vi "Contact closure.vi"(0 "Task In CC":refnum<k21>) -> ()   [LabVIEW 2016]
uses:
  <vilib>/Utility/error.llb/DialogType.ctl
  <vilib>/DAQmx/write.llb/DAQmx Write (Analog DBL 1Chan 1Samp).vi
  <vilib>/DAQmx/miscellaneous.llb/DAQmx Fill In Error Info.vi
  Utility/Global_Laser.vi
  Utility/Global Constants.vi
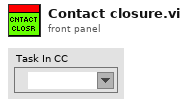
[diagram p1: front panel]
types:
  T1 = typedef "DialogType.ctl" = u16
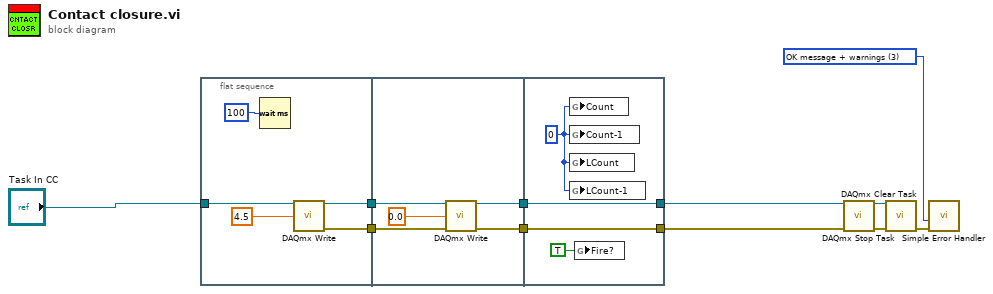
[diagram p0: block diagram]
diagram:
  w6 = T1 3 items=["no dialog", "OK message", "continue or stop message", "OK message + warnings", "continue/stop + warnings"] ("type of dialog (OK msg:1)")
  n1 = flat-sequence {
    tunnel: [w16] -> w5
    tunnel: [w15] -> w4
    tunnel: "Task In CC" -> [w12]
    tunnel: w5 -> [w21]
    tunnel: w4 -> [w19]
    tunnel: [w20] -> w3
    tunnel: [w18] -> w2
    tunnel: [w24] -> w10
    tunnel: [w25] -> w9
    tunnel: w3 -> [w25]
    tunnel: w2 -> [w24]
    frame #0 {
      n2 = Wait (ms)(milliseconds to wait=u32 100 ("millisecond multiple")) -> ()  [unwired: 1 out]
      n3 = call-poly <vilib>:"DAQmx Write.vi"("task/channels in"=w12, "data"=4.5) -> ("task out"=w15:refnum<k21>, "error out"=w16:errorcluster)  [unwired: 11 in, 1 out]
    }
    frame #1 {
      n4 = call-poly <vilib>:"DAQmx Write.vi"("task/channels in"=w19, "data"=0.0, "error in"=w21) -> ("task out"=w18:refnum<k21>, "error out"=w20:errorcluster)  [unwired: 10 in, 1 out]
    }
    frame #2 {
      w23 = u32 0
      n5 = global write "Global Constants.vi" "Count"(w23) -> ()
      n6 = global write "Global Constants.vi" "Count-1"(w23) -> ()
      n7 = global write "Global_Laser.vi" "LCount"(w23) -> ()
      n8 = global write "Global_Laser.vi" "LCount-1"(w23) -> ()
      n9 = global write "Global_Laser.vi" "Fire?"(TRUE ("Fire?")) -> ()
    }
  }
  n10 = call <vilib>:"DAQmx Stop Task.vi"("task/channels in"=w10, "error in"=w9) -> ("task out"=w8:refnum<k21>, "error out"=w7:errorcluster)  [unwired: 12 in]
  n11 = call <vilib>:"DAQmx Clear Task.vi"("task in"=w8, "error in"=w7) -> ("error out"=w11:errorcluster)  [unwired: 13 in]
  n12 = call <vilib>:"Simple Error Handler.vi"("type of dialog (OK msg:1)"=w6, "error in (no error)"=w11) -> ()  [unwired: 3 in, 5 out]
